vi "CalibrateIntegrationTime.vi"(8 "error in (no error)":errorcluster, 11 "Instruments in":refnum<class "Instruments.lvclass">) -> (0 "error out":errorcluster, 3 "Instruments out":refnum<class "Instruments.lvclass">)   [LabVIEW 2012, in "Instruments.lvclass"]
uses:
  Instruments.lvclass
  Controls/Config.ctl
  Instruments.lvclass/Instruments.ctl
  SpectrumCommands.ctl
  Controls/SpectrometerOphirSelector.ctl
  SpectrumWindowExit.vi
panel:
  out "max value 2":dbl
  out "max value":dbl
  out "Target":bool
  out "Saturated":bool
  out "DeviceIndicator":bool
  in  "TurnOffDevice":bool
  in  "TurnOnDevice":bool
  in  "TestType":enum16{"Disabled", "Calibrate", "Continuous"}(ring)
  out "Vf":dbl format="%0.2f"
  out "Keithley":refnum<visa-resource-name>
  in  "Graph":cluster{"Y":dbl[], "Y":dbl[]}[](graph)
  in  "Int Time, Final":i32
  in  "Calibrate":bool
  out "Ready":bool
  in  "Int Time(ms)":i32
  in  "Enabled":bool
  in  "Exit":bool
  in  "StopCapture":bool
  in  "StartCapture":bool
  # "Instructions:\n1: Press start capture\n2: Adjust integration time until spectrum is visible\n3: Press calibrate integration\n4: When calibration finished press Exit"
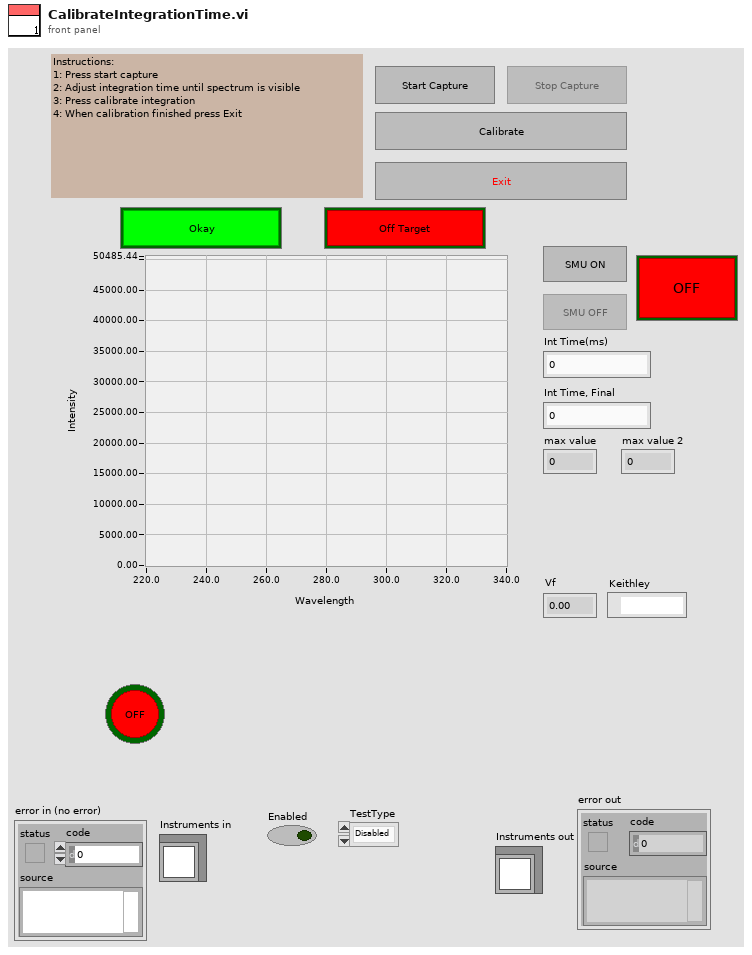
[diagram p1: front panel]
types:
  T1 = enum8{"Enabled", "Disabled", "Disabled and Grayed Out"}
  T2 = cluster{"StopCapture":refnum<vi>, "StartCapture":refnum<vi>, "Exit":refnum<vi>, "Enabled":refnum<vi>, "Ready":refnum<vi>, "Calibrate":refnum<vi>, "TurnOnDevice":refnum<vi>, "TurnOffDevice":refnum<vi>}
  T3 = typedef "Config.ctl" = cluster{"IntTime":i32, "Samples":i32, "PowerMin":dbl, "KneeMin":dbl, "KneeMax":dbl, "Background Wl":dbl, "Settle Delay,ms":u32, "StationId":sgl}
  T4 = typedef "SpectrumCommands.ctl" = enum16{"Init", "StartCapture", "StopCapture", "Calibrate", "TurnDeviceOn", "TurnOffDevice", "Exit"}
  T5 = typedef "SpectrometerOphirSelector.ctl" = enum16{"Get Background", "Measure", "Measure50", "Raw"}
  T6 = cluster{"Wavelength":dbl[], "EL Spectrum":dbl[]}[]
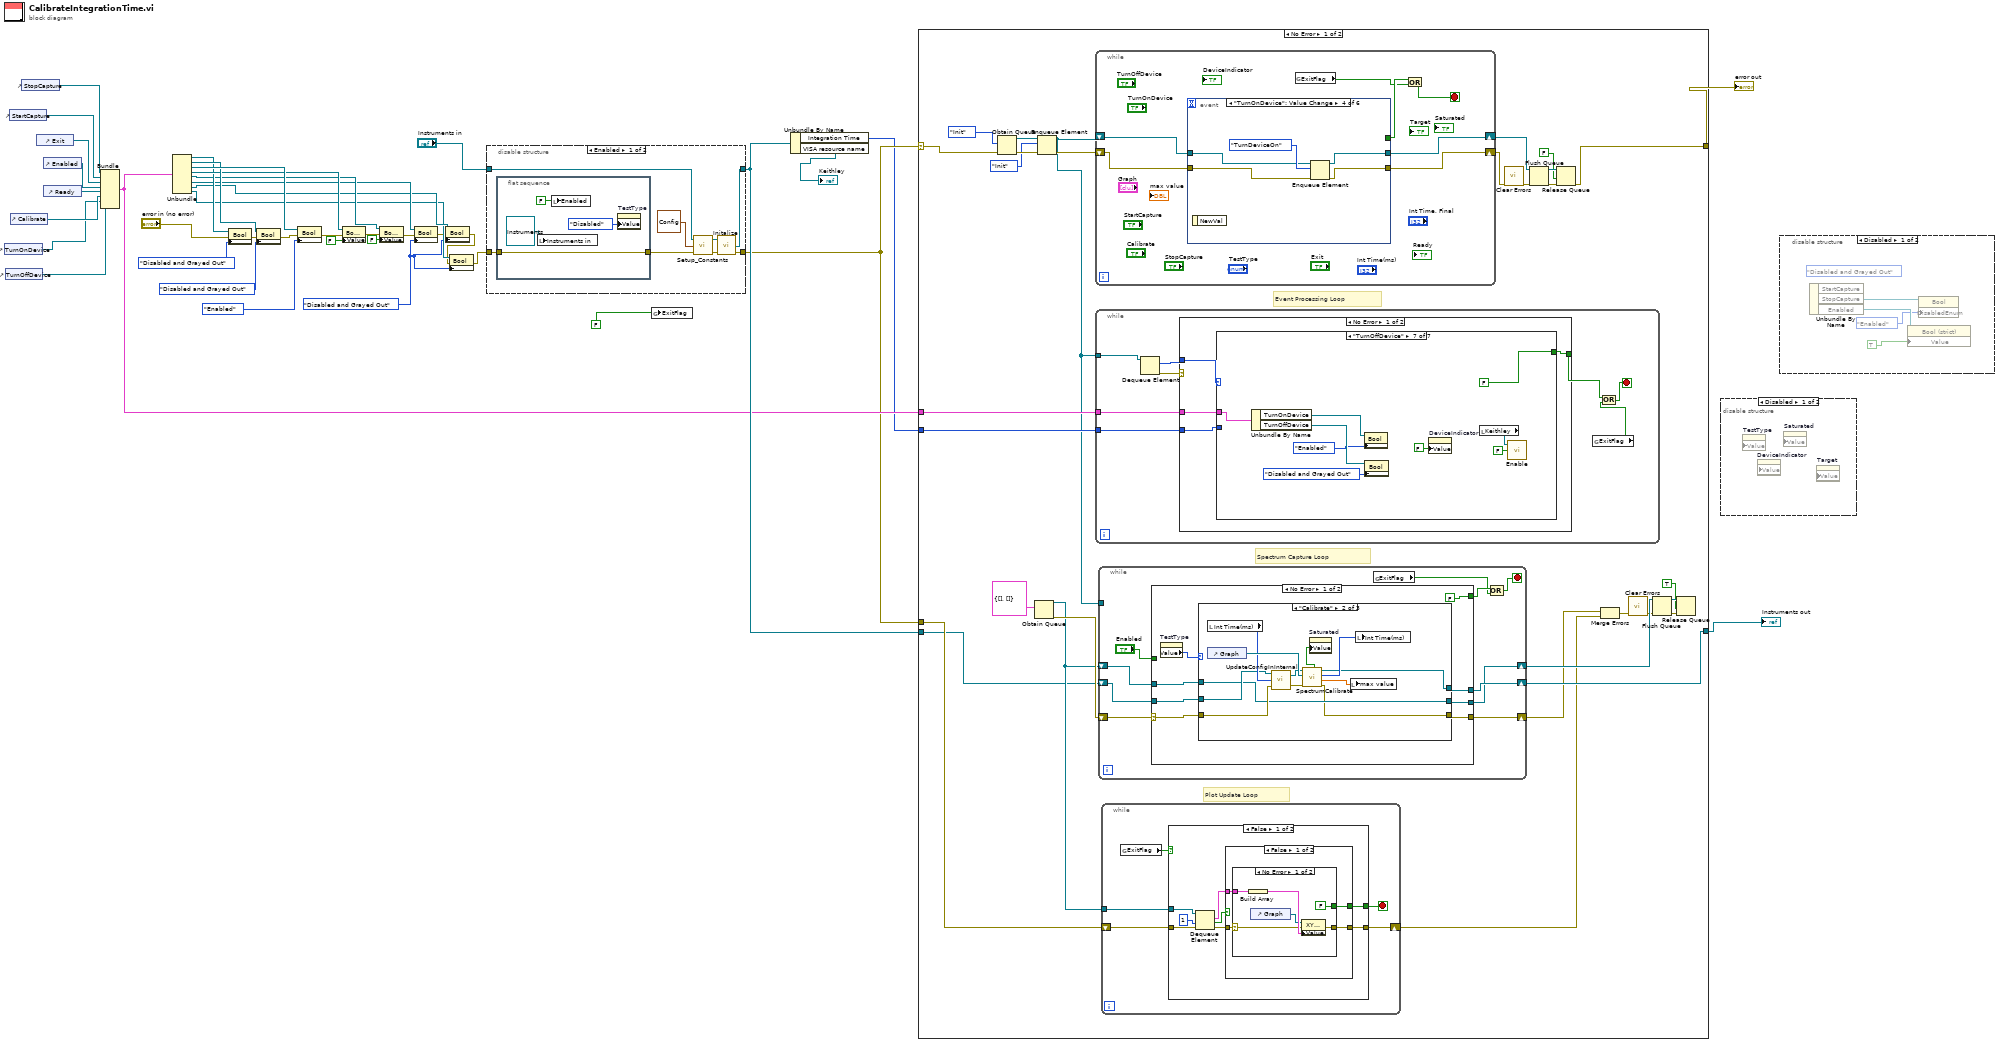
[diagram p0: block diagram]
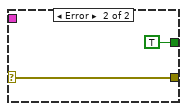
[diagram p5: hidden frame]
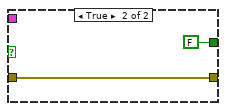
[diagram p6: hidden frame]
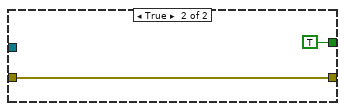
[diagram p7: hidden frame]
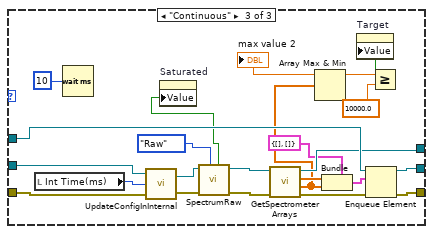
[diagram p9: hidden frame]
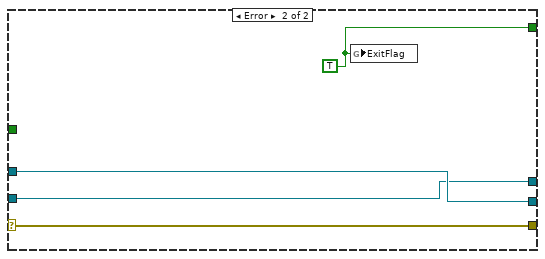
[diagram p10: hidden frame]
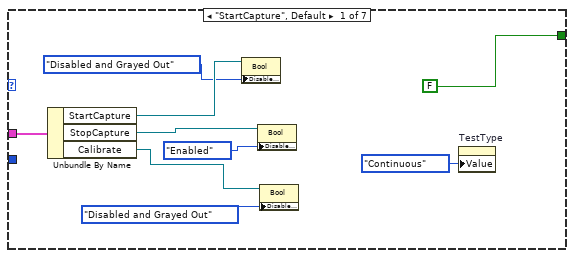
[diagram p11: hidden frame]
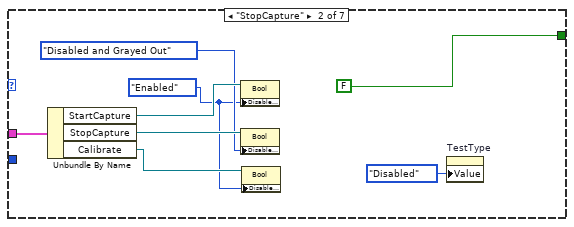
[diagram p12: hidden frame]
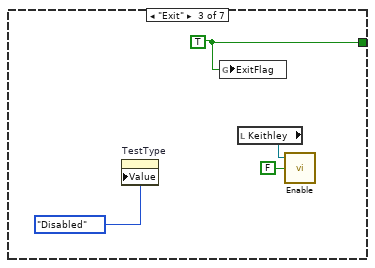
[diagram p13: hidden frame]
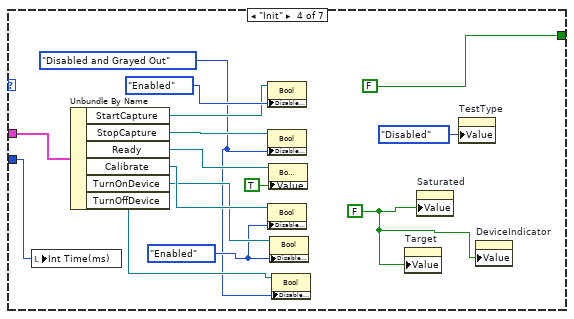
[diagram p14: hidden frame]
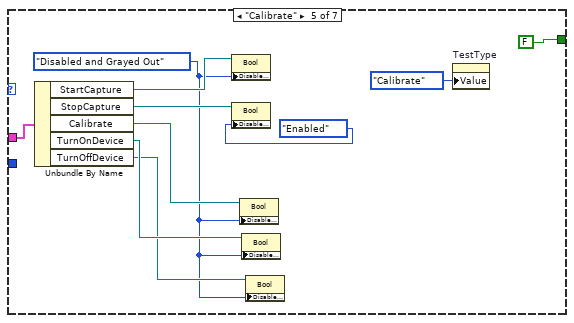
[diagram p15: hidden frame]
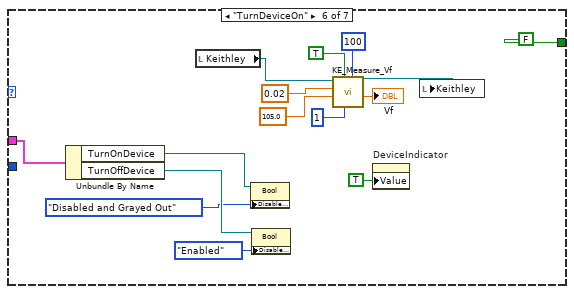
[diagram p16: hidden frame]
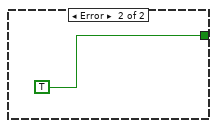
[diagram p17: hidden frame]
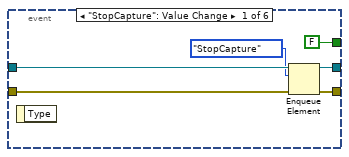
[diagram p18: hidden frame]
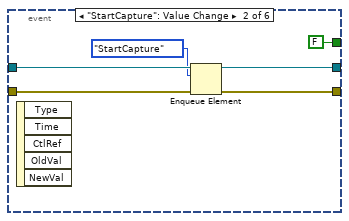
[diagram p19: hidden frame]
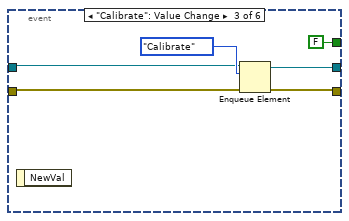
[diagram p20: hidden frame]
diagram:
  w5 = T1."Disabled and Grayed Out" ("Disabled")
  n1 = control-ref of="TurnOnDevice"() -> (w14:refnum<vi>)
  n2 = control-ref of="TurnOffDevice"() -> (w13:refnum<vi>)
  n3 = control-ref of="StartCapture"() -> (w37:refnum<vi>)
  n4 = control-ref of="Calibrate"() -> (w15:refnum<vi>)
  n5 = control-ref of="StopCapture"() -> (w38:refnum<vi>)
  n6 = control-ref of="Exit"() -> (w36:refnum<vi>)
  n7 = control-ref of="Enabled"() -> (w35:refnum<vi>)
  n8 = control-ref of="Ready"() -> (w32:refnum<vi>)
  n9 = Bundle("StopCapture"=w38, "StartCapture"=w37, "Exit"=w36, "Enabled"=w35, "Ready"=w32, "Calibrate"=w15, "TurnOnDevice"=w14, "TurnOffDevice"=w13) -> (w20:T2)  [unwired: 1 in]
  n10 = Unbundle(w20) -> ("StopCapture"=w25:refnum<vi>, "StartCapture"=w29:refnum<vi>, "Exit"=w31:refnum<vi>, "Enabled"=w27:refnum<vi>, "Ready"=w12:refnum<vi>, "Calibrate"=w11:refnum<vi>, "TurnOnDevice"=w10:refnum<vi>, "TurnOffDevice"=w9:refnum<vi>)
  n11 = property class="Bool"(reference=w25, error in="error in (no error)", "DisabledEnum"=T1."Disabled and Grayed Out" ("Disabled")) -> (error out=w23:errorcluster)  [unwired: 1 out]
  n12 = property class="Bool"(reference=w29, error in=w23, "DisabledEnum"=T1."Disabled and Grayed Out" ("Disabled")) -> (error out=w22:errorcluster)  [unwired: 1 out]
  n13 = property class="Bool"(reference=w31, error in=w22, "DisabledEnum"=T1."Enabled" ("Disabled")) -> (error out=w21:errorcluster)  [unwired: 1 out]
  n14 = property class="Bool (strict)"(reference=w27, error in=w21, "Value"=FALSE) -> (error out=w8:errorcluster)  [unwired: 1 out]
  n15 = property class="Bool (strict)"(reference=w12, error in=w8, "Value"=FALSE) -> (error out=w3:errorcluster)  [unwired: 1 out]
  n16 = property class="Bool"(reference=w11, error in=w3, "DisabledEnum"=w5) -> (error out=w4:errorcluster)  [unwired: 1 out]
  n17 = property class="Bool"(reference=w10, error in=w4, "DisabledEnum"=w5) -> (error out=w2:errorcluster)  [unwired: 1 out]
  n18 = property class="Bool"(reference=w9, error in=w2, "DisabledEnum"=w5) -> (error out=w1:errorcluster)  [unwired: 1 out]
  n19 = disable-structure shown="Enabled" {
    disable-tunnel: [w48 w53] -> w33
    disable-tunnel: [w47 w54] -> w19
    disable-tunnel: "Instruments in" -> [w43 w53]
    disable-tunnel: w1 -> [w41 w54]
    frame Enabled {
      n20 = flat-sequence {
        tunnel: [w51] -> w42
        tunnel: w41 -> [w51]
        frame #0 {
          n21 = local write "Instruments in"(refnum<class "Instruments.lvclass"> refnum ("Instruments in")) -> ()
          n22 = local write "Enabled"(FALSE ("Enabled")) -> ()
          n23 = property on="TestType" class="Enum (strict)"("Value"=enum16{"Disabled", "Calibrate", "Continuous"}."Disabled" ("TestType")) -> ()  [unwired: 2 in, 2 out]
        }
      }
      n24 = call-dynamic "Setup_Constants.vi"("error in (no error)"=w42, "Config In"=T3 {"IntTime"=100, "Samples"=3, "PowerMin"=300.0, "KneeMin"=-20.0, "KneeMax"=20.0, "Background Wl"=275.0, "Settle Delay,ms"=0, "StationId"=0.0}, "Instruments in"=w43) -> ("error out"=w44:errorcluster, "Instruments out"=w45:refnum<class "Instruments.lvclass">)  [unwired: 1 in]
      n25 = call-dynamic "Initalize.vi"("error in (no error)"=w44, "Instruments in"=w45) -> ("error out"=w47:errorcluster, "Instruments out"=w48:refnum<class "Instruments.lvclass">)  [unwired: 2 in]
    }
    frame Disabled {
    }
  }
  n26 = global write "SpectrumWindowExit.vi" "ExitFlag"(FALSE ("Enabled")) -> ()
  n27 = Unbundle By Name(w33) -> ("Integration Time"=w16:i32, "VISA resource name"=→"Keithley":refnum<visa-resource-name>)
  n28 = case shown="No Error" w19 {
    selector: w19 -> [w83 w298]
    tunnel: [w74 w298] -> w40
    tunnel: [w80 w297] -> w39
    tunnel: w33 -> [w56 w297]
    tunnel: w20 -> [w57 _]
    tunnel: w19 -> [w78 _]
    tunnel: w16 -> [w58 _]
    frame No Error {
      # "Spectrum Capture Loop"
      # "Plot Update Loop"
      # "Event Processing Loop"
      n29 = Obtain Queue(element data type=SpectrumCommands."Init", error in (no error)=w83) -> (queue out=w62:refnum<queue>, error out=w61:errorcluster)  [unwired: 3 in, 1 out]
      n30 = Obtain Queue(element data type=cluster{"Wavelength":dbl[], "EL Spectrum":dbl[]} {"Wavelength"=[], "EL Spectrum"=[]}) -> (queue out=w79:refnum<queue>, error out=w81:errorcluster)  [unwired: 4 in, 1 out]
      n31 = Enqueue Element(queue=w62, element=SpectrumCommands."Init", error in (no error)=w61) -> (queue out=w55:refnum<queue>, error out=w59:errorcluster)  [unwired: 1 in, 1 out]
      n32 = while {
        shift-right: [w259] -> w75
        shift-left: w55 -> [w262]
        shift-right: [w260] -> w68
        shift-left: w59 -> [w261]
        stop <- w257 stop-if-true
        n33 = event shown="[3] \"TurnOnDevice\": Value Change" {
          selector: _ -> [_ _ _ _ _ _]
          dyn-events: _ -> [_ _ _ _ _ _]
          timeout: _ -> [_ _ _ _ _ _]
          tunnel: w262 -> [w268 w274 w279 w284 w289 w296]
          tunnel: w261 -> [w267 w273 w278 w283 w290 w295]
          tunnel: [w266 w272 w277 w282 w286 w294] -> w260
          tunnel: [w265 w271 w276 w281 w287 w293] -> w259
          tunnel: [FALSE ("ExitFlag") FALSE ("ExitFlag") FALSE ("ExitFlag") _ _ TRUE ("ExitFlag")] -> w258
          event "StopCapture": Value Change {
            n34 = event-data() -> ()  [unwired: 1 in, 1 out]
            n35 = Enqueue Element(queue=w268, element=SpectrumCommands."StopCapture", error in (no error)=w267) -> (queue out=w265:refnum<queue>, error out=w266:errorcluster)  [unwired: 1 in, 1 out]
          }
          event "StartCapture": Value Change {
            n36 = event-data() -> ()  [unwired: 1 in, 5 out]
            n37 = Enqueue Element(queue=w274, element=SpectrumCommands."StartCapture", error in (no error)=w273) -> (queue out=w271:refnum<queue>, error out=w272:errorcluster)  [unwired: 1 in, 1 out]
          }
          event "Calibrate": Value Change {
            n38 = event-data() -> ()  [unwired: 1 in, 1 out]
            n39 = Enqueue Element(queue=w279, element=SpectrumCommands."Calibrate", error in (no error)=w278) -> (queue out=w276:refnum<queue>, error out=w277:errorcluster)  [unwired: 1 in, 1 out]
          }
          event "TurnOnDevice": Value Change {
            n40 = event-data() -> ()  [unwired: 1 in, 1 out]
            n41 = Enqueue Element(queue=w284, element=SpectrumCommands."TurnDeviceOn", error in (no error)=w283) -> (queue out=w281:refnum<queue>, error out=w282:errorcluster)  [unwired: 1 in, 1 out]
          }
          event "TurnOffDevice": Value Change {
            n42 = event-data() -> ()  [unwired: 1 in, 1 out]
            n43 = Enqueue Element(queue=w289, element=SpectrumCommands."TurnOffDevice", error in (no error)=w290) -> (queue out=w287:refnum<queue>, error out=w286:errorcluster)  [unwired: 1 in, 1 out]
          }
          event "Exit": Value Change {
            n44 = event-data() -> ()  [unwired: 1 in, 1 out]
            n45 = Enqueue Element(queue=w296, element=SpectrumCommands."Exit", error in (no error)=w295) -> (queue out=w293:refnum<queue>, error out=w294:errorcluster)  [unwired: 1 in, 1 out]
          }
        }
        n46 = global read "SpectrumWindowExit.vi" "ExitFlag"() -> (w256:bool)
        n47 = Or(x=w258, y=w256) -> (x .or. y?=w257:bool)
      }
      n48 = while {
        tunnel: w57 -> [w178]
        tunnel: w58 -> [w174]
        tunnel: w55 -> [w173]
        stop <- w176 stop-if-true
        n49 = Dequeue Element(queue=w173) -> (element=w179:T4, error out=w180:errorcluster)  [unwired: 2 in, 2 out]
        n50 = case shown="No Error" w180 {
          tunnel: w179 -> [w184 _]
          tunnel: w178 -> [w183 _]
          tunnel: [w182 TRUE ("x")] -> w177
          tunnel: w174 -> [w181 _]
          frame No Error {
            n51 = case shown="\"TurnOffDevice\"" w184 {
              tunnel: w183 -> [w193 w199 _ w216 w227 w236 w247]
              tunnel: [FALSE ("x") FALSE ("x") w205 FALSE ("x") FALSE ("x") FALSE ("x") FALSE ("x")] -> w182
              tunnel: w181 -> [_ _ _ w219 _ _ _]
              frame "StartCapture", Default {
                n52 = Unbundle By Name(w193) -> ("StartCapture"=w192:refnum<vi>, "StopCapture"=w190:refnum<vi>, "Calibrate"=w185:refnum<vi>)
                n53 = property class="Bool"(reference=w192, "DisabledEnum"=T1."Disabled and Grayed Out" ("Disabled")) -> ()  [unwired: 1 in, 2 out]
                n54 = property class="Bool"(reference=w190, "DisabledEnum"=T1."Enabled" ("Disabled")) -> ()  [unwired: 1 in, 2 out]
                n55 = property class="Bool"(reference=w185, "DisabledEnum"=T1."Disabled and Grayed Out" ("Disabled")) -> ()  [unwired: 1 in, 2 out]
                n56 = property on="TestType" class="Enum (strict)"("Value"=enum16{"Disabled", "Calibrate", "Continuous"}."Continuous" ("TestType")) -> ()  [unwired: 2 in, 2 out]
              }
              frame "StopCapture" {
                w194 = T1."Enabled" ("Disabled")
                n57 = Unbundle By Name(w199) -> ("StartCapture"=w201:refnum<vi>, "StopCapture"=w200:refnum<vi>, "Calibrate"=w195:refnum<vi>)
                n58 = property class="Bool"(reference=w201, "DisabledEnum"=w194) -> ()  [unwired: 1 in, 2 out]
                n59 = property class="Bool"(reference=w200, "DisabledEnum"=T1."Disabled and Grayed Out" ("Disabled")) -> ()  [unwired: 1 in, 2 out]
                n60 = property class="Bool"(reference=w195, "DisabledEnum"=w194) -> ()  [unwired: 1 in, 2 out]
                n61 = property on="TestType" class="Enum (strict)"("Value"=enum16{"Disabled", "Calibrate", "Continuous"}."Disabled" ("TestType")) -> ()  [unwired: 2 in, 2 out]
              }
              frame "Exit" {
                w205 = TRUE ("x")
                n62 = property on="TestType" class="Enum (strict)"("Value"=enum16{"Disabled", "Calibrate", "Continuous"}."Disabled" ("TestType")) -> ()  [unwired: 2 in, 2 out]
                n63 = global write "SpectrumWindowExit.vi" "ExitFlag"(w205) -> ()
                n64 = local read "Keithley"() -> (w204:refnum<visa-resource-name>)
                n65 = call "Enable.vi"("Enable Output (T: Enable)"=FALSE, "VISA resource name"=w204) -> ()  [unwired: 1 in, 2 out]
              }
              frame "Init" {
                w206 = FALSE ("Saturated")
                w208 = T1."Enabled" ("Disabled")
                w207 = T1."Disabled and Grayed Out" ("Disabled")
                n66 = local write "Int Time(ms)"(w219) -> ()
                n67 = Unbundle By Name(w216) -> ("StartCapture"=w214:refnum<vi>, "StopCapture"=w218:refnum<vi>, "Ready"=w213:refnum<vi>, "Calibrate"=w211:refnum<vi>, "TurnOnDevice"=w210:refnum<vi>, "TurnOffDevice"=w209:refnum<vi>)
                n68 = property class="Bool"(reference=w214, "DisabledEnum"=T1."Enabled" ("Disabled")) -> ()  [unwired: 1 in, 2 out]
                n69 = property class="Bool"(reference=w218, "DisabledEnum"=w207) -> ()  [unwired: 1 in, 2 out]
                n70 = property class="Bool"(reference=w211, "DisabledEnum"=w208) -> ()  [unwired: 1 in, 2 out]
                n71 = property class="Bool (strict)"(reference=w213, "Value"=TRUE) -> ()  [unwired: 1 in, 2 out]
                n72 = property class="Bool"(reference=w210, "DisabledEnum"=w208) -> ()  [unwired: 1 in, 2 out]
                n73 = property class="Bool"(reference=w209, "DisabledEnum"=w207) -> ()  [unwired: 1 in, 2 out]
                n74 = property on="Target" class="Bool (strict)"("Value"=w206) -> ()  [unwired: 2 in, 2 out]
                n75 = property on="Saturated" class="Bool (strict)"("Value"=w206) -> ()  [unwired: 2 in, 2 out]
                n76 = property on="TestType" class="Enum (strict)"("Value"=enum16{"Disabled", "Calibrate", "Continuous"}."Disabled" ("TestType")) -> ()  [unwired: 2 in, 2 out]
                n77 = property on="DeviceIndicator" class="Bool (strict)"("Value"=w206) -> ()  [unwired: 2 in, 2 out]
              }
              frame "Calibrate" {
                w222 = T1."Disabled and Grayed Out" ("Disabled")
                n78 = Unbundle By Name(w227) -> ("StartCapture"=w230:refnum<vi>, "StopCapture"=w229:refnum<vi>, "Calibrate"=w225:refnum<vi>, "TurnOnDevice"=w224:refnum<vi>, "TurnOffDevice"=w223:refnum<vi>)
                n79 = property class="Bool"(reference=w230, "DisabledEnum"=w222) -> ()  [unwired: 1 in, 2 out]
                n80 = property class="Bool"(reference=w229, "DisabledEnum"=T1."Enabled" ("Disabled")) -> ()  [unwired: 1 in, 2 out]
                n81 = property class="Bool"(reference=w225, "DisabledEnum"=w222) -> ()  [unwired: 1 in, 2 out]
                n82 = property class="Bool"(reference=w224, "DisabledEnum"=w222) -> ()  [unwired: 1 in, 2 out]
                n83 = property class="Bool"(reference=w223, "DisabledEnum"=w222) -> ()  [unwired: 1 in, 2 out]
                n84 = property on="TestType" class="Enum (strict)"("Value"=enum16{"Disabled", "Calibrate", "Continuous"}."Calibrate" ("TestType")) -> ()  [unwired: 2 in, 2 out]
              }
              frame "TurnDeviceOn" {
                n85 = Unbundle By Name(w236) -> ("TurnOnDevice"=w235:refnum<vi>, "TurnOffDevice"=w234:refnum<vi>)
                n86 = local read "Keithley"() -> (w245:refnum<visa-resource-name>)
                n87 = property class="Bool"(reference=w235, "DisabledEnum"=T1."Disabled and Grayed Out" ("Disabled")) -> ()  [unwired: 1 in, 2 out]
                n88 = property class="Bool"(reference=w234, "DisabledEnum"=T1."Enabled" ("Disabled")) -> ()  [unwired: 1 in, 2 out]
                n89 = call "KE_Measure_Vf.vi"("Settle Delay"=u32 100, "Samples"=1, "Keep On"=TRUE, "Compliance"=105.0, "Current(A)"=0.02, "KE_In"=w245) -> ("Vf"=→"Vf":dbl, "KE_Out"=w238:refnum<visa-resource-name>)  [unwired: 3 in, 1 out]
                n90 = property on="DeviceIndicator" class="Bool (strict)"("Value"=TRUE ("DeviceIndicator")) -> ()  [unwired: 2 in, 2 out]
                n91 = local write "Keithley"(w238) -> ()
              }
              frame "TurnOffDevice" {
                n92 = Unbundle By Name(w247) -> ("TurnOnDevice"=w251:refnum<vi>, "TurnOffDevice"=w250:refnum<vi>)
                n93 = property class="Bool"(reference=w251, "DisabledEnum"=T1."Enabled" ("Disabled")) -> ()  [unwired: 1 in, 2 out]
                n94 = property class="Bool"(reference=w250, "DisabledEnum"=T1."Disabled and Grayed Out" ("Disabled")) -> ()  [unwired: 1 in, 2 out]
                n95 = property on="DeviceIndicator" class="Bool (strict)"("Value"=FALSE ("DeviceIndicator")) -> ()  [unwired: 2 in, 2 out]
                n96 = local read "Keithley"() -> (w254:refnum<visa-resource-name>)
                n97 = call "Enable.vi"("Enable Output (T: Enable)"=FALSE, "VISA resource name"=w254) -> ()  [unwired: 1 in, 2 out]
              }
            }
          }
          frame Error {
          }
        }
        n98 = global read "SpectrumWindowExit.vi" "ExitFlag"() -> (w175:bool)
        n99 = Or(x=w177, y=w175) -> (x .or. y?=w176:bool)
      }
      n100 = while {
        shift-right: [w119] -> w69
        shift-left: w79 -> [w120]
        shift-right: [w121] -> w80
        shift-left: w56 -> [w122]
        shift-right: [w118] -> w66
        shift-left: w81 -> [w117]
        tunnel: w55 -> [_]
        stop <- w114 stop-if-true
        n101 = case shown="No Error" w117 {
          selector: w117 -> [w126 w170]
          tunnel: "Enabled" -> [_ _]
          tunnel: w122 -> [w131 w171]
          tunnel: [w130 w171] -> w121
          tunnel: w120 -> [w129 w172]
          tunnel: [w128 w172] -> w119
          tunnel: [w127 w170] -> w118
          tunnel: [FALSE ("ExitFlag") w169] -> w116
          frame No Error {
            n102 = property on="TestType" class="Enum (strict)"() -> ("Value"=w124:enum16{"Disabled", "Calibrate", "Continuous"})  [unwired: 2 in, 2 out]
            n103 = case shown="\"Calibrate\"" w124 {
              tunnel: w131 -> [w133 w144 w159]
              tunnel: [w133 w139 w165] -> w130
              tunnel: w129 -> [w134 w138 w168]
              tunnel: [w134 w138 w166] -> w128
              tunnel: [w132 w137 w163] -> w127
              tunnel: w126 -> [w132 w143 w157]
              frame "Disabled", Default {
              }
              frame "Calibrate" {
                n104 = local read "Int Time(ms)"() -> (w145:i32)
                n105 = control-ref of="Graph"() -> (w146:refnum<vi>)
                n106 = call-dynamic "UpdateConfigInInternal.vi"("error in (no error)"=w143, "IntTime"=w145, "Instruments in"=w144) -> ("error out"=w142:errorcluster, "Instruments out"=w141:refnum<class "Instruments.lvclass">)
                n107 = call-dynamic "SpectrumCalibrate.vi"("error in (no error)"=w142, "Graph In"=w146, "Instruments in"=w141) -> ("error out"=w137:errorcluster, "max value"=w135:dbl, "Integration Time"=w140:i32, "Instruments out"=w139:refnum<class "Instruments.lvclass">, "In Range?"=w136:bool)  [unwired: 3 in, 1 out]
                n108 = property on="Saturated" class="Bool (strict)"("Value"=w136) -> ()  [unwired: 2 in, 2 out]
                n109 = local write "max value"(w135) -> ()
                n110 = local write "Int Time(ms)"(w140) -> ()
              }
              frame "Continuous" {
                n111 = local read "Int Time(ms)"() -> (w158:i32)
                n112 = Wait (ms)(milliseconds to wait=u32 10) -> ()  [unwired: 1 out]
                n113 = call-dynamic "UpdateConfigInInternal.vi"("error in (no error)"=w157, "IntTime"=w158, "Instruments in"=w159) -> ("error out"=w155:errorcluster, "Instruments out"=w156:refnum<class "Instruments.lvclass">)
                n114 = call-dynamic "SpectrumRaw.vi"("Type"=SpectrometerOphirSelector."Raw", "error in (no error)"=w155, "Instruments in"=w156) -> ("error out"=w154:errorcluster, "Instruments out"=w153:refnum<class "Instruments.lvclass">, "Saturated?"=w151:bool)  [unwired: 4 in, 2 out]
                n115 = property on="Saturated" class="Bool (strict)"("Value"=w151) -> ()  [unwired: 2 in, 2 out]
                n116 = call-dynamic "GetSpectrometerArrays.vi"("error in (no error)"=w154, "Instruments in"=w153) -> ("error out"=w164:errorcluster, "Spectrum"=w150:dbl[], "Wavelength"=w160:dbl[], "Instruments out"=w165:refnum<class "Instruments.lvclass">)  [unwired: 6 in]
                n117 = Array Max & Min(array=w150) -> (max value=w149:dbl)  [unwired: 3 out]
                "max value 2" <- w149
                n118 = Bundle(cluster=cluster{"Wavelength":dbl[], "EL Spectrum":dbl[]} {"Wavelength"=[], "EL Spectrum"=[]}, "Wavelength"=w160, "EL Spectrum"=w150) -> (w167:cluster{"Wavelength":dbl[], "EL Spectrum":dbl[]})
                n119 = Enqueue Element(queue=w168, element=w167, error in (no error)=w164) -> (queue out=w166:refnum<queue>, error out=w163:errorcluster)  [unwired: 1 in, 1 out]
                n120 = Greater Or Equal?(x=w149, y=10000.0) -> (x >= y?=w147:bool)
                n121 = property on="Target" class="Bool (strict)"("Value"=w147) -> ()  [unwired: 2 in, 2 out]
              }
            }
          }
          frame Error {
            w169 = TRUE ("ExitFlag")
            n122 = global write "SpectrumWindowExit.vi" "ExitFlag"(w169) -> ()
          }
        }
        n123 = global read "SpectrumWindowExit.vi" "ExitFlag"() -> (w115:bool)
        n124 = Or(x=w116, y=w115) -> (x .or. y?=w114:bool)
      }
      n125 = while {
        tunnel: w79 -> [w85]
        shift-right: [w89] -> w65
        shift-left: w78 -> [w87]
        stop <- w86 stop-if-true
        n126 = global read "SpectrumWindowExit.vi" "ExitFlag"() -> (w88:bool)
        n127 = case shown="False" w88 {
          tunnel: [w95 w113] -> w89
          tunnel: w87 -> [w92 w113]
          tunnel: [w94 TRUE] -> w86
          tunnel: w85 -> [w93 _]
          frame False {
            n128 = Dequeue Element(queue=w93, timeout in ms (-1)=1, error in (no error)=w92) -> (element=w96:cluster{"Wavelength":dbl[], "EL Spectrum":dbl[]}, timed out?=w90:bool, error out=w97:errorcluster)  [unwired: 1 out]
            n129 = case shown="False" w90 {
              tunnel: w97 -> [w101 w111]
              tunnel: w96 -> [w100 _]
              tunnel: [w99 w111] -> w95
              tunnel: [w98 FALSE] -> w94
              frame False {
                n130 = case shown="No Error" w101 {
                  selector: w101 -> [w104 w108]
                  tunnel: w100 -> [w107 _]
                  tunnel: [FALSE TRUE] -> w98
                  tunnel: [w103 w108] -> w99
                  frame No Error {
                    n131 = Build Array(w107) -> (w105:T6)
                    n132 = control-ref of="Graph"() -> (w102:refnum<vi>)
                    n133 = property class="XYGraph (strict)"(reference=w102, error in=w104, "Value"=w105) -> (error out=w103:errorcluster)  [unwired: 1 out]
                  }
                  frame Error {
                  }
                }
              }
              frame True {
              }
            }
          }
          frame True {
          }
        }
      }
      n134 = call <vilib>:"Clear Errors.vi"("error in (no error)"=w68) -> ("error out"=w67:errorcluster)  [unwired: 6 in]
      n135 = Flush Queue(queue=w75, error in (no error)=w67) -> (queue out=w77:refnum<queue>, error out=w76:errorcluster)  [unwired: 1 out]
      n136 = Release Queue(queue=w77, force destroy? (F)=FALSE, error in (no error)=w76) -> (error out=w74:errorcluster)  [unwired: 2 out]
      n137 = Merge Errors(w66, w65) -> (w64:errorcluster)
      n138 = call <vilib>:"Clear Errors.vi"("error in (no error)"=w64) -> ("error out"=w63:errorcluster)  [unwired: 6 in]
      n139 = Flush Queue(queue=w69, error in (no error)=w63) -> (queue out=w72:refnum<queue>, error out=w71:errorcluster)  [unwired: 1 out]
      n140 = Release Queue(queue=w72, force destroy? (F)=TRUE, error in (no error)=w71) -> ()  [unwired: 3 out]
    }
    frame Error {
    }
  }
  "error out" <- w40
  "Instruments out" <- w39
  n141 = disable-structure shown="Disabled" {
    frame Disabled {
      n142 = property on="TestType" class="Enum (strict)" props=["Value"]() -> ()  [unwired: 3 in, 2 out]
      n143 = property on="DeviceIndicator" class="Bool (strict)" props=["Value"]() -> ()  [unwired: 3 in, 2 out]
      n144 = property on="Saturated" class="Bool (strict)" props=["Value"]() -> ()  [unwired: 3 in, 2 out]
      n145 = property on="Target" class="Bool (strict)" props=["Value"]() -> ()  [unwired: 3 in, 2 out]
    }
    frame Enabled {
    }
  }
  n146 = disable-structure shown="Disabled" {
    frame Disabled {
      w300 = T1."Disabled and Grayed Out" ("Disabled")
      n147 = Unbundle By Name() -> ("StartCapture"=w299:refnum<vi>, "StopCapture"=w301:refnum<vi>, "Enabled"=w303:refnum<vi>)  [unwired: 1 in]
      n148 = property class="Bool (strict)"(reference=w303, "Value"=TRUE) -> ()  [unwired: 1 in, 2 out]
      n149 = property class="Bool"(reference=w301, "DisabledEnum"=T1."Enabled" ("Disabled")) -> ()  [unwired: 1 in, 2 out]
    }
    frame Enabled {
    }
  }
